vi "R5_Control.vi"() -> ()   [LabVIEW 2016]
uses:
  LabviewBioreactor/Reactor Control/R3R4/R2 example/R2 DO Manual Control.ctl
  LabviewBioreactor/Reactor Control/R3R4/R2 example/R2 Pump Manual Control.ctl
  LabviewBioreactor/Reactor Control/R3R4/R2 example/R2 pH Manual Control.ctl
  LabviewBioreactor/Reactor Control/R3R4/R2 example/R2 Reactor Status v1.ctl
  LabviewBioreactor/Reactor Control/R3R4/R2 example/R2Variables.lvlib
  LabviewBioreactor/Reactor Control/R3R4/R2 example/R2 SBR Mode Control.ctl
  R2 example/R2 Cycle Status.ctl
panel:
  out "Elapsed Time":dbl
  in  "Aerobic DO Control":T1={"DO set point (mg/L)"=2.0, "N2 Gain"=35.0, "Air Gain"=15.0, "DO Tolerance (mg/L)"=0.1, "Air Short Reaction Time (s)"=60.0, "Long Reaction Time (s)"=90.0, "N2 Short Reaction Time (s) 2"=15.0}
  out "pH and DO":cluster{"pH":dbl, "DO (mg/L)":dbl}(graph)
  out "DO Intercept":dbl
  out "DO Slope":dbl
  out "pH Intercept":dbl
  out "pH Slope":dbl
  in  "DO Control":T2
  in  "Reactor 2 Pumps Manual Control":T3
  in  "pH Control":T4
  in  "pH Control":T5={" pH Set Point"=7.5, " pH Tolerance"=0.1, "Reaction Time (s)"=15.0, "Pump On Time (s)"=3.0}
  out "Cycle Phase":T6 max=5.0 scale=0.0..160.0
  in  "SBR Timing":T7={"Anaerobic Time (min)"=60.0, "Aerobic (min)"=240.0, "Settle 1"=3.0, "Decant 1 (min)"=5.0, "Mix 2"=0.0, "Idle Time (min)"=5.0, "Aerobic no DO control (min)"=2.0, "Settle 2 (min)"=0.0, "Decant 2 (min)"=0.0, "Mix 3"=0.0, "Settle 3"=0.0, "Decant 3"=0.0}
  out "N2 and Air Flow":cluster{"N2 Flow":dbl, "Air Flow":dbl}(graph)
  out "Reactor 2 Status":T8 {"Compressed Air" format="%#.0g"; "Release Flow" format="%#.0g"; "DO Amp (A)" format="%#.4g"; "pH Amp (A)" format="%#.4g"; "DO (mg/L)" format="%#.2g"; "pH" format="%#.2g"}
  in  "Pumps Manual Control":bool
  in  "DO Manual Control":bool
  in  "pH Manual Control":bool=TRUE
  in  "DO Calibrate":bool
  in  "pH Calibrate":bool
  # "On: Manual Mode\nOff: SBR Mode"
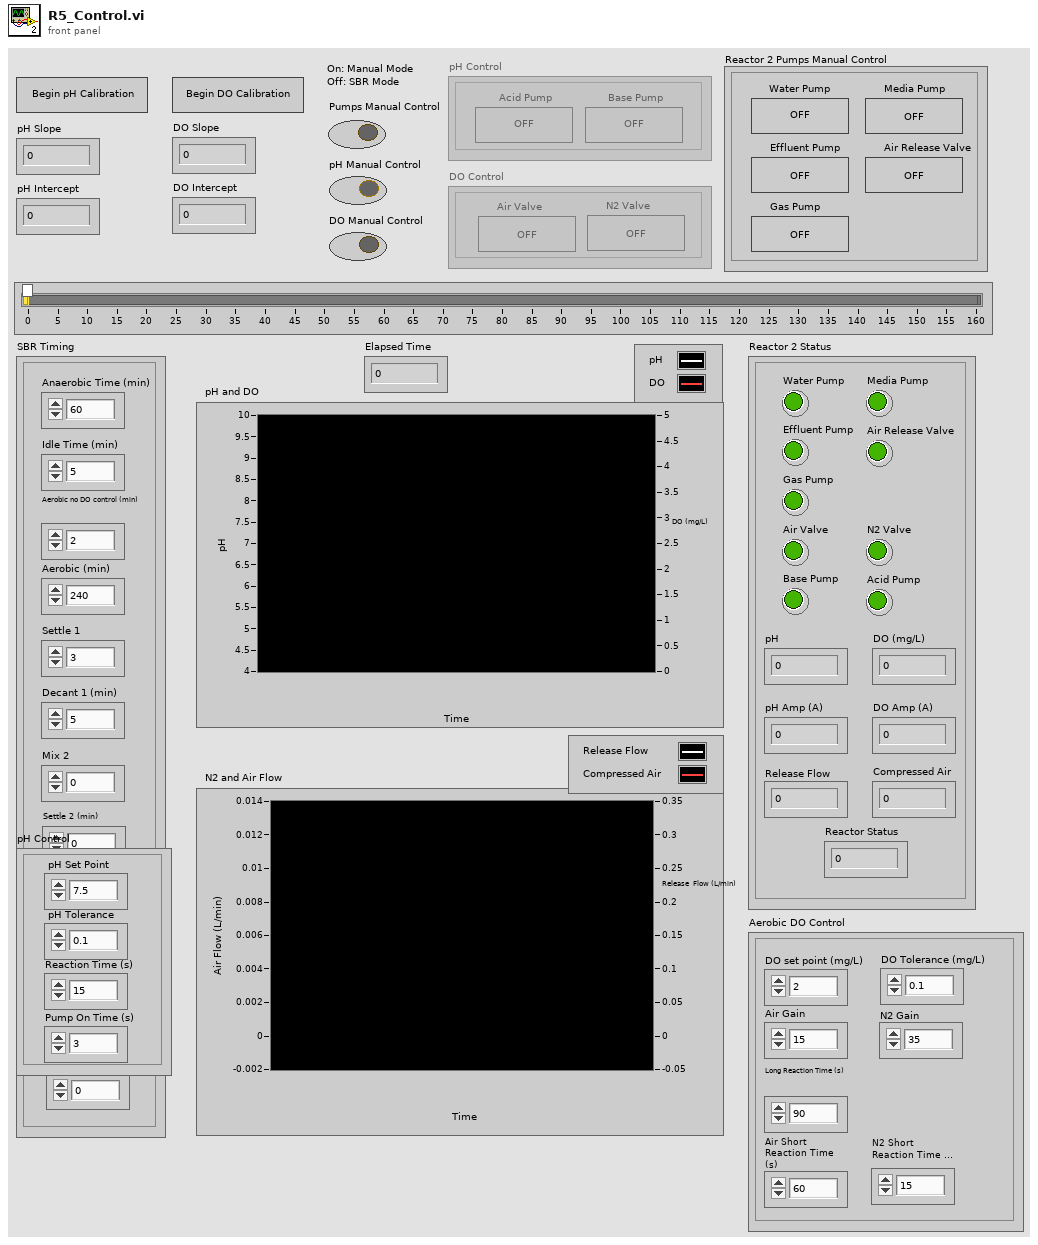
[diagram p1: front panel]
types:
  T1 = cluster{"DO set point (mg/L)":dbl, "N2 Gain":dbl, "Air Gain":dbl, "DO Tolerance (mg/L)":dbl, "Air Short Reaction Time (s)":dbl, "Long Reaction Time (s)":dbl, "N2 Short Reaction Time (s) 2":dbl}
  T2 = typedef "R2 DO Manual Control.ctl" = cluster{"Air Valve":bool, "N2 Valve":bool}
  T3 = typedef "R2Variables.lvlib/R2 Pump Manual Control.ctl" = cluster{"Water Pump":bool, "Effluent Pump":bool, "Media Pump":bool, "Gas Pump":bool, "Air Release Valve":bool}
  T4 = typedef "R2Variables.lvlib/R2 pH Manual Control.ctl" = cluster{"Acid Pump":bool, "Base Pump":bool}
  T5 = cluster{" pH Set Point":dbl, " pH Tolerance":dbl, "Reaction Time (s)":dbl, "Pump On Time (s)":dbl}
  T6 = typedef "R2Variables.lvlib/R2 Cycle Status.ctl" = dbl
  T7 = typedef "R2Variables.lvlib/R2 SBR Mode Control.ctl" = cluster{"Anaerobic Time (min)":dbl, "Aerobic (min)":dbl, "Settle 1":dbl, "Decant 1 (min)":dbl, "Mix 2":dbl, "Idle Time (min)":dbl, "Aerobic no DO control (min)":dbl, "Settle 2 (min)":dbl, "Decant 2 (min)":dbl, "Mix 3":dbl, "Settle 3":dbl, "Decant 3":dbl}
  T8 = typedef "R2Variables.lvlib/R2 Reactor Status v1.ctl" = cluster{"Water Pump":bool, "Media Pump":bool, "Effluent Pump":bool, "Base Pump":bool, "Gas Pump":bool, "Acid Pump":bool, "Air Release Valve":bool, "N2 Valve":bool, "pH":dbl, "DO (mg/L)":dbl, "pH Amp (A)":dbl, "DO Amp (A)":dbl, "Release Flow":dbl, "Compressed Air":dbl, "Reactor Status":sgl, "Air Valve":bool}
  T9 = enum8{"Enabled", "Disabled", "Disabled and Grayed Out"}
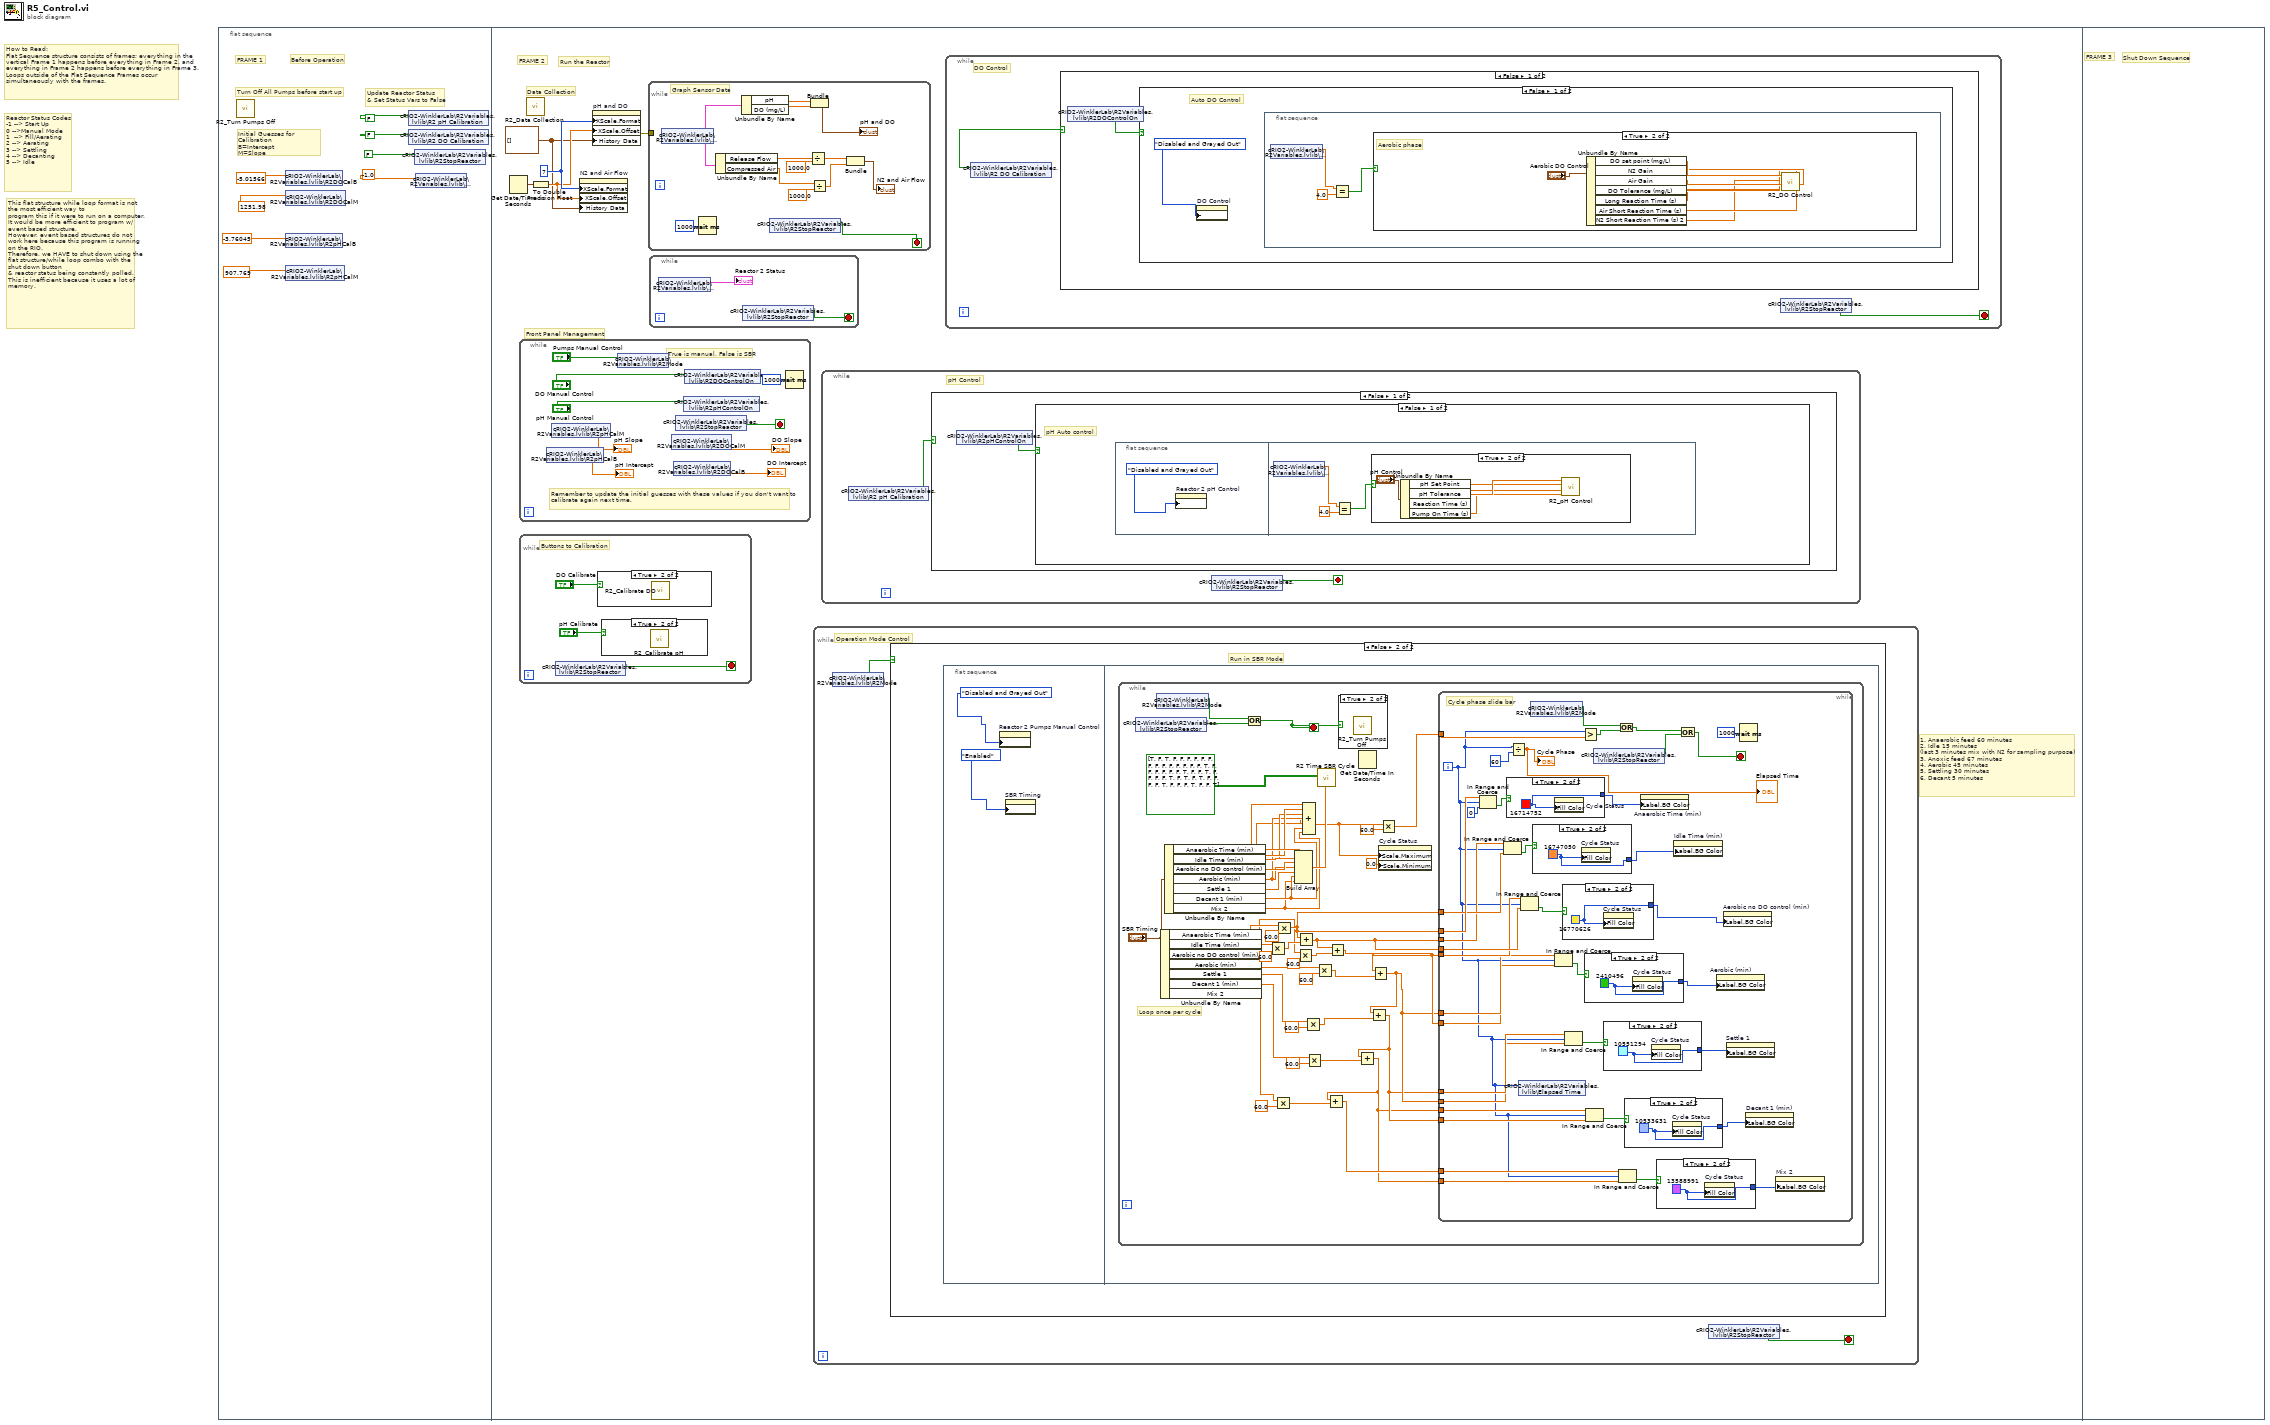
[diagram p0: block diagram]
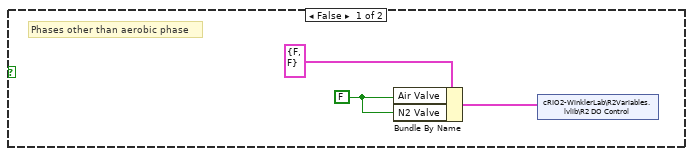
[diagram p2: hidden frame]
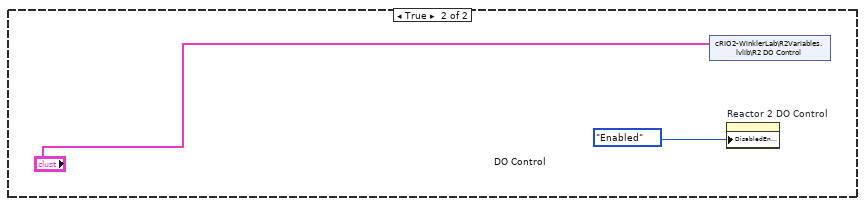
[diagram p3: hidden frame]
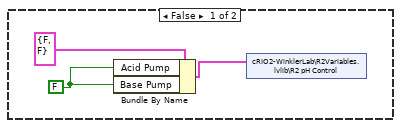
[diagram p7: hidden frame]
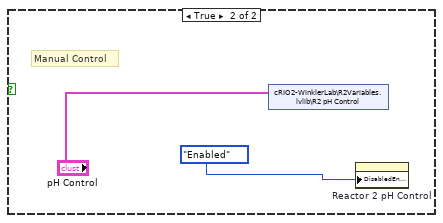
[diagram p8: hidden frame]
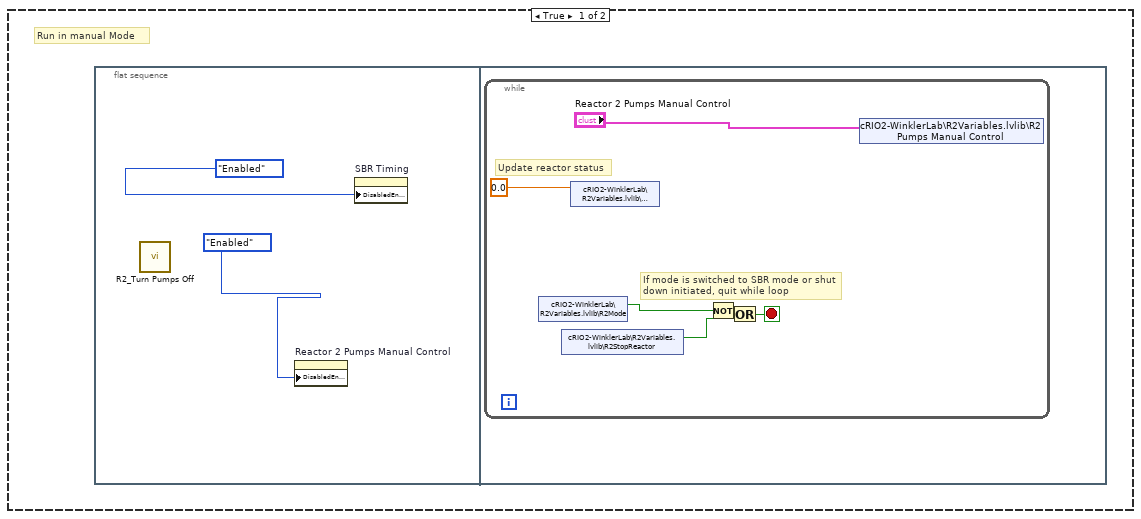
[diagram p10: hidden frame]
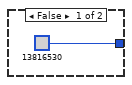
[diagram p11: hidden frame]
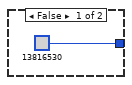
[diagram p12: hidden frame]
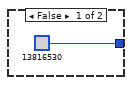
[diagram p13: hidden frame]
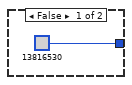
[diagram p14: hidden frame]
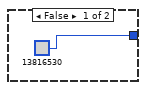
[diagram p15: hidden frame]
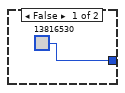
[diagram p16: hidden frame]
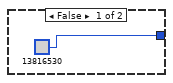
[diagram p17: hidden frame]
diagram:
  # "Reactor Status Codes\n-1 --> Start Up\n0 -->Manual Mode\n1  --> Fill/Aerating\n2 --> Aerating\n3 --> Settling\n4 --> Decanting\n5 --> Idle"
  # "How to Read:\nFlat Sequence structure consists of frames; everything in the vertical Frame 1 happens before everything in Frame 2, and everything in Frame 2 happens before everything in Frame 3.\nLoops outside of the Flat Sequence Frames occur simultaneously with the frames."
  # "This flat structure while loop format is not the most efficient way to \nprogram this if it were to run on a computer.\nIt would be more efficient to program w/ event based structure.\nHowever, event based structures do not work here because this program is running on the RIO.\nTherefore, we HAVE to shut down using the flat structure/while loop combo with the shut down button \n& reactor status being constantly polled.\nThis is inefficient because it uses a lot of memory."
  n1 = flat-sequence {
    frame #0 {
      # "Initial Guesses for Calibration\nB=Intercept\nM=Slope"
      # "Update Reactor Status \n& Set Status Vars to False"
      # "Turn Off All Pumps before start up"
      # "FRAME 1"
      # "Before Operation"
      n2 = call "R2_Turn Pumps Off.vi"() -> ()  [unwired: 12 in]
      n3 = shared-variable "cRIO2-WinklerLab\\R2Variables.lvlib\\R2DOCalB"(-5.01566 ("R1DOxCalB")) -> ()  [unwired: 1 in, 1 out]
      n4 = shared-variable "cRIO2-WinklerLab\\R2Variables.lvlib\\R2DOCalM"(1251.98 ("R1DOxCalM")) -> ()  [unwired: 1 in, 1 out]
      n5 = shared-variable "cRIO2-WinklerLab\\R2Variables.lvlib\\R2pHCalB"(-3.76045 ("R1pHCalB")) -> ()  [unwired: 1 in, 1 out]
      n6 = shared-variable "cRIO2-WinklerLab\\R2Variables.lvlib\\R2pHCalM"(907.769 ("R1pHCalM")) -> ()  [unwired: 1 in, 1 out]
      n7 = shared-variable "cRIO2-WinklerLab\\R2Variables.lvlib\\R2 pH Calibration"(FALSE ("pH Calibration")) -> ()  [unwired: 1 in, 1 out]
      n8 = shared-variable "cRIO2-WinklerLab\\R2Variables.lvlib\\R2 DO Calibration"(FALSE ("DO Calibration")) -> ()  [unwired: 1 in, 1 out]
      n9 = shared-variable "cRIO2-WinklerLab\\R2Variables.lvlib\\R2StopReactor"(FALSE ("R1Stop Reactor")) -> ()  [unwired: 1 in, 1 out]
      n10 = shared-variable "cRIO2-WinklerLab\\R2Variables.lvlib\\R2Phase"(-1.0) -> ()  [unwired: 1 in, 1 out]
    }
    frame #1 {
      w9 = cluster{"pH":dbl, "DO (mg/L)":dbl}[] [] ("History Data")
      w11 = u8 7 ("X Scale.Display Format:Format")
      # "1. Anaerobic feed 60 minutes\n2. Idle 15 minutes \n(last 3 minutes mix with N2 for sampling purpose)\n3. Anoxic feed 67 minutes\n4. Aerobic 45 minutes\n5. Settling 30 minutes\n6. Decant 5 minutes"
      # "Front Panel Management"
      # "Data Collection"
      # "FRAME 2"
      # "Run the Reactor"
      n11 = Get Date/Time In Seconds() -> (seconds since 1Jan1904=w13:timestamp)
      n12 = while {
        stop <- w73 stop-if-true
        # "Remember to update the initial guesses with these values if you don't want to calibrate again next time."
        # "True is manual, False is SBR"
        n13 = shared-variable "cRIO2-WinklerLab\\R2Variables.lvlib\\R2pHCalB"() -> (→"pH Intercept":dbl)  [unwired: 1 in, 1 out]
        n14 = shared-variable "cRIO2-WinklerLab\\R2Variables.lvlib\\R2pHCalM"() -> (→"pH Slope":dbl)  [unwired: 1 in, 1 out]
        n15 = shared-variable "cRIO2-WinklerLab\\R2Variables.lvlib\\R2Mode"("Pumps Manual Control") -> ()  [unwired: 1 in, 1 out]
        n16 = shared-variable "cRIO2-WinklerLab\\R2Variables.lvlib\\R2DOCalM"() -> (→"DO Slope":dbl)  [unwired: 1 in, 1 out]
        n17 = shared-variable "cRIO2-WinklerLab\\R2Variables.lvlib\\R2DOCalB"() -> (→"DO Intercept":dbl)  [unwired: 1 in, 1 out]
        n18 = shared-variable "cRIO2-WinklerLab\\R2Variables.lvlib\\R2StopReactor"() -> (w73:bool)  [unwired: 1 in, 1 out]
        n19 = shared-variable "cRIO2-WinklerLab\\R2Variables.lvlib\\R2pHControlOn"("pH Manual Control") -> ()  [unwired: 1 in, 1 out]
        n20 = shared-variable "cRIO2-WinklerLab\\R2Variables.lvlib\\R2DOControlOn"("DO Manual Control") -> ()  [unwired: 1 in, 1 out]
        n21 = Wait (ms)(milliseconds to wait=u32 1000) -> ()  [unwired: 1 out]
      }
      n22 = while {
        stop <- w49 stop-if-true
        # "Buttons to Calibration"
        n23 = shared-variable "cRIO2-WinklerLab\\R2Variables.lvlib\\R2StopReactor"() -> (w49:bool)  [unwired: 1 in, 1 out]
        n24 = case shown="True" "DO Calibrate" {
          frame False {
          }
          frame True {
            n25 = call "R2_Calibrate DO.vi"() -> ()  [unwired: 12 in]
          }
        }
        n26 = case shown="True" "pH Calibrate" {
          frame False {
          }
          frame True {
            n27 = call "R2_Calibrate pH.vi"() -> ()  [unwired: 12 in]
          }
        }
      }
      n28 = call "R2_Data Collection.vi"() -> ()  [unwired: 12 in]
      n29 = To Double Precision Float(number=w13) -> (double precision float=w10:dbl)
      n30 = property on="N2 and Air Flow" class="WFChart (strict)"("XScale.Format"=w11, "XScale.Offset"=w10, "History Data"=w9) -> ()  [unwired: 2 in, 2 out]
      n31 = property on="pH and DO" class="WFChart (strict)"("XScale.Format"=w11, "XScale.Offset"=w10, "History Data"=w9) -> (error out=w12:errorcluster)  [unwired: 2 in, 1 out]
      n32 = while {
        tunnel: w12 -> [_]
        stop <- w24 stop-if-true
        # "Graph Sensor Data"
        n33 = shared-variable "cRIO2-WinklerLab\\R2Variables.lvlib\\R2Status"() -> (w25:T8)  [unwired: 1 in, 1 out]
        n34 = Wait (ms)(milliseconds to wait=u32 1000) -> ()  [unwired: 1 out]
        n35 = Unbundle By Name(w25) -> ("Release Flow"=w21:dbl, "Compressed Air"=w18:dbl)
        n36 = Unbundle By Name(w25) -> ("pH"=w26:dbl, "DO (mg/L)"=w27:dbl)
        n37 = shared-variable "cRIO2-WinklerLab\\R2Variables.lvlib\\R2StopReactor"() -> (w24:bool)  [unwired: 1 in, 1 out]
        n38 = Divide(x=w21, y=1000.0) -> (x/y=w17:dbl)
        n39 = Bundle("pH"=w26, "DO (mg/L)"=w27) -> (→"pH and DO":cluster{"pH":dbl, "DO (mg/L)":dbl})  [unwired: 1 in]
        n40 = Divide(x=w18, y=1000.0) -> (x/y=w16:dbl)
        n41 = Bundle(w17, w16) -> (→"N2 and Air Flow":cluster{dbl, dbl})  [unwired: 1 in]
      }
      n42 = while {
        stop <- w14 stop-if-true
        n43 = shared-variable "cRIO2-WinklerLab\\R2Variables.lvlib\\R2Status"() -> (→"Reactor 2 Status":T8)  [unwired: 1 in, 1 out]
        n44 = shared-variable "cRIO2-WinklerLab\\R2Variables.lvlib\\R2StopReactor"() -> (w14:bool)  [unwired: 1 in, 1 out]
      }
      n45 = while {
        stop <- w79 stop-if-true
        # "Operation Mode Control"
        n46 = shared-variable "cRIO2-WinklerLab\\R2Variables.lvlib\\R2Mode"() -> (w78:bool)  [unwired: 1 in, 1 out]
        n47 = case shown="False" w78 {
          frame True {
            # "Run in manual Mode"
            n48 = flat-sequence {
              frame #0 {
                n49 = call "R2_Turn Pumps Off.vi"() -> ()  [unwired: 12 in]
                n50 = property on="Reactor 2 Pumps Manual Control" class="Clust (strict)"("DisabledEnum"=T9."Enabled" ("Disabled")) -> ()  [unwired: 2 in, 2 out]
                n51 = property on="SBR Timing" class="Clust (strict)"("DisabledEnum"=T9."Enabled" ("Disabled")) -> ()  [unwired: 2 in, 2 out]
              }
              frame #1 {
                n52 = while {
                  stop <- w86 stop-if-true
                  # "If mode is switched to SBR mode or shut \ndown initiated, quit while loop"
                  # "Update reactor status"
                  n53 = shared-variable "cRIO2-WinklerLab\\R2Variables.lvlib\\R2Mode"() -> (w84:bool)  [unwired: 1 in, 1 out]
                  n54 = shared-variable "cRIO2-WinklerLab\\R2Variables.lvlib\\R2StopReactor"() -> (w83:bool)  [unwired: 1 in, 1 out]
                  n55 = shared-variable "cRIO2-WinklerLab\\R2Variables.lvlib\\R2Phase"(0.0 ("Reactor Status")) -> ()  [unwired: 1 in, 1 out]
                  n56 = Not(x=w84) -> (.not. x?=w87:bool)
                  n57 = Or(x=w87, y=w83) -> (x .or. y?=w86:bool)
                  n58 = shared-variable "cRIO2-WinklerLab\\R2Variables.lvlib\\R2 Pumps Manual Control"("Reactor 2 Pumps Manual Control") -> ()  [unwired: 1 in, 1 out]
                }
              }
            }
          }
          frame False {
            # "Run in SBR Mode"
            n59 = flat-sequence {
              frame #0 {
                n60 = property on="Reactor 2 Pumps Manual Control" class="Clust (strict)"("DisabledEnum"=T9."Disabled and Grayed Out" ("Disabled")) -> ()  [unwired: 2 in, 2 out]
                n61 = property on="SBR Timing" class="Clust (strict)"("DisabledEnum"=T9."Enabled" ("Disabled")) -> ()  [unwired: 2 in, 2 out]
              }
              frame #1 {
                n62 = while {
                  stop <- w133 stop-if-true
                  # "Loop once per cycle"
                  n63 = shared-variable "cRIO2-WinklerLab\\R2Variables.lvlib\\R2StopReactor"() -> (w131:bool)  [unwired: 1 in, 1 out]
                  n64 = shared-variable "cRIO2-WinklerLab\\R2Variables.lvlib\\R2Mode"() -> (w132:bool)  [unwired: 1 in, 1 out]
                  n65 = Unbundle By Name("SBR Timing") -> ("Anaerobic Time (min)"=w118:dbl, "Idle Time (min)"=w113:dbl, "Aerobic no DO control (min)"=w111:dbl, "Aerobic (min)"=w109:dbl, "Settle 1"=w105:dbl, "Decant 1 (min)"=w98:dbl, "Mix 2"=w93:dbl)
                  n66 = Unbundle By Name("SBR Timing") -> ("Anaerobic Time (min)"=w129:dbl, "Idle Time (min)"=w128:dbl, "Aerobic no DO control (min)"=w127:dbl, "Aerobic (min)"=w126:dbl, "Settle 1"=w125:dbl, "Decant 1 (min)"=w100:dbl, "Mix 2"=w90:dbl)
                  n67 = Or(x=w132, y=w131) -> (x .or. y?=w133:bool)
                  n68 = Multiply(x=w113, y=60.0) -> (x*y=w112:dbl)
                  n69 = Multiply(x=w93, y=60.0) -> (x*y=w94:dbl)
                  n70 = Multiply(x=w118, y=60.0) -> (x*y=w117:dbl)
                  n71 = Build Array(w129, w128, w127, w126, w125, w100, w90) -> (w124:dbl[])
                  n72 = Multiply(x=w111, y=60.0) -> (x*y=w110:dbl)
                  n73 = Add(x=w117, y=w112) -> (x+y=w119:dbl)
                  n74 = Compound Arithmetic op=ADD(w129, w128, w127, w126, w125, w100, w90) -> (w120:dbl)
                  n75 = Multiply(x=w105, y=60.0) -> (x*y=w104:dbl)
                  n76 = Multiply(x=w98, y=60.0) -> (x*y=w97:dbl)
                  n77 = Multiply(x=w109, y=60.0) -> (x*y=w103:dbl)
                  n78 = call "R2 Time SBR Cycle.vi"("Pump Status Array"=bool[][] [[TRUE, FALSE, TRUE, FALSE, FALSE, FALSE, FALSE], [FALSE, FALSE, FALSE, FALSE, FALSE, FALSE, FALSE], [FALSE, FALSE, FALSE, TRUE, FALSE, FALSE, FALSE], [FALSE, FALSE, FALSE, TRUE, FALSE, FALSE, TRUE], [FALSE, FALSE, FALSE, FALSE, TRUE, FALSE, TRUE], [FALSE, TRUE, FALSE, FALSE, FALSE, FALSE, TRUE], [FALSE, FALSE, FALSE, TRUE, FALSE, FALSE, TRUE]], "Timing Array"=w124) -> ()  [unwired: 10 in]
                  n79 = Add(x=w119, y=w110) -> (x+y=w102:dbl)
                  n80 = case shown="True" w133 {
                    frame False {
                    }
                    frame True {
                      n81 = call "R2_Turn Pumps Off.vi"() -> ()  [unwired: 12 in]
                    }
                  }
                  n82 = Get Date/Time In Seconds() -> ()  [unwired: 1 out]
                  n83 = Add(x=w102, y=w103) -> (x+y=w101:dbl)
                  n84 = Add(x=w101, y=w104) -> (x+y=w96:dbl)
                  n85 = Add(x=w96, y=w97) -> (x+y=w91:dbl)
                  n86 = Add(x=w91, y=w94) -> (x+y=w92:dbl)
                  n87 = property on="Cycle Status" class="Slide (strict)"("Scale.Maximum"=w120, "Scale.Minimum"=0.0 ("Scale.Range:Minimum")) -> ()  [unwired: 2 in, 2 out]
                  n88 = Multiply(x=w120, y=60.0) -> (x*y=w121:dbl)
                  n89 = while {
                    tunnel: w121 -> [w170]
                    tunnel: w117 -> [w165]
                    tunnel: w117 -> [w162]
                    tunnel: w119 -> [w161]
                    tunnel: w119 -> [w160]
                    tunnel: w102 -> [w159]
                    tunnel: w101 -> [w158]
                    tunnel: w96 -> [w151]
                    tunnel: w101 -> [w150]
                    tunnel: w102 -> [w148]
                    tunnel: w91 -> [w146]
                    tunnel: w96 -> [w145]
                    tunnel: w92 -> [w143]
                    tunnel: w91 -> [w142]
                    i -> [w141]
                    stop <- w152 stop-if-true
                    # "Cycle phase slide bar"
                    n90 = In Range and Coerce(upper limit=w165, x=w141, lower limit=0) -> (In Range?=w168:bool)  [unwired: 1 out]
                    n91 = In Range and Coerce(upper limit=w161, x=w141, lower limit=w162) -> (In Range?=w166:bool)  [unwired: 1 out]
                    n92 = case shown="True" w168 {
                      tunnel: [u32 13816530 w185] -> w157
                      frame False {
                      }
                      frame True {
                        w185 = u32 16714752
                        n93 = property on="Cycle Status" class="Slide (strict)"("Fill Color"=w185) -> ()  [unwired: 2 in, 2 out]
                      }
                    }
                    n94 = Divide(x=w141, y=60) -> (x/y=→"Cycle Phase" →"Elapsed Time":dbl)
                    n95 = shared-variable "cRIO2-WinklerLab\\R2Variables.lvlib\\Elapsed Time"(w141) -> ()  [unwired: 1 in, 1 out]
                    n96 = In Range and Coerce(upper limit=w159, x=w141, lower limit=w160) -> (In Range?=w164:bool)  [unwired: 1 out]
                    n97 = shared-variable "cRIO2-WinklerLab\\R2Variables.lvlib\\R2Mode"() -> (w155:bool)  [unwired: 1 in, 1 out]
                    n98 = case shown="True" w166 {
                      tunnel: [u32 13816530 w183] -> w140
                      frame False {
                      }
                      frame True {
                        w183 = u32 16747050
                        n99 = property on="Cycle Status" class="Slide (strict)"("Fill Color"=w183) -> ()  [unwired: 2 in, 2 out]
                      }
                    }
                    n100 = In Range and Coerce(upper limit=w158, x=w141, lower limit=w148) -> (In Range?=w163:bool)  [unwired: 1 out]
                    n101 = case shown="True" w164 {
                      tunnel: [u32 13816530 w181] -> w135
                      frame False {
                      }
                      frame True {
                        w181 = u32 16770626
                        n102 = property on="Cycle Status" class="Slide (strict)"("Fill Color"=w181) -> ()  [unwired: 2 in, 2 out]
                      }
                    }
                    n103 = In Range and Coerce(upper limit=w151, x=w141, lower limit=w150) -> (In Range?=w149:bool)  [unwired: 1 out]
                    n104 = Greater?(x=w141, y=w170) -> (0:w156:bool)
                    n105 = case shown="True" w163 {
                      tunnel: [u32 13816530 w179] -> w139
                      frame False {
                      }
                      frame True {
                        w179 = u32 2410496
                        n106 = property on="Cycle Status" class="Slide (strict)"("Fill Color"=w179) -> ()  [unwired: 2 in, 2 out]
                      }
                    }
                    n107 = In Range and Coerce(upper limit=w146, x=w141, lower limit=w145) -> (In Range?=w147:bool)  [unwired: 1 out]
                    n108 = shared-variable "cRIO2-WinklerLab\\R2Variables.lvlib\\R2StopReactor"() -> (w153:bool)  [unwired: 1 in, 1 out]
                    n109 = case shown="True" w149 {
                      tunnel: [u32 13816530 w177] -> w138
                      frame False {
                      }
                      frame True {
                        w177 = u32 10551294
                        n110 = property on="Cycle Status" class="Slide (strict)"("Fill Color"=w177) -> ()  [unwired: 2 in, 2 out]
                      }
                    }
                    n111 = Or(x=w155, y=w156) -> (x .or. y?=w154:bool)
                    n112 = In Range and Coerce(upper limit=w143, x=w141, lower limit=w142) -> (In Range?=w144:bool)  [unwired: 1 out]
                    n113 = case shown="True" w147 {
                      tunnel: [u32 13816530 w175] -> w137
                      frame False {
                      }
                      frame True {
                        w175 = u32 10533631
                        n114 = property on="Cycle Status" class="Slide (strict)"("Fill Color"=w175) -> ()  [unwired: 2 in, 2 out]
                      }
                    }
                    n115 = property on="Anaerobic Time (min)" class="DigNum (strict)"("Label.BG Color"=w157) -> ()  [unwired: 2 in, 2 out]
                    n116 = case shown="True" w144 {
                      tunnel: [u32 13816530 w173] -> w136
                      frame False {
                      }
                      frame True {
                        w173 = u32 13588991
                        n117 = property on="Cycle Status" class="Slide (strict)"("Fill Color"=w173) -> ()  [unwired: 2 in, 2 out]
                      }
                    }
                    n118 = property on="Idle Time (min)" class="DigNum (strict)"("Label.BG Color"=w140) -> ()  [unwired: 2 in, 2 out]
                    n119 = Or(x=w154, y=w153) -> (x .or. y?=w152:bool)
                    n120 = property on="Aerobic (min)" class="DigNum (strict)"("Label.BG Color"=w139) -> ()  [unwired: 2 in, 2 out]
                    n121 = property on="Aerobic no DO control (min)" class="DigNum (strict)"("Label.BG Color"=w135) -> ()  [unwired: 2 in, 2 out]
                    n122 = property on="Settle 1" class="DigNum (strict)"("Label.BG Color"=w138) -> ()  [unwired: 2 in, 2 out]
                    n123 = Wait (ms)(milliseconds to wait=u32 1000) -> ()  [unwired: 1 out]
                    n124 = property on="Decant 1 (min)" class="DigNum (strict)"("Label.BG Color"=w137) -> ()  [unwired: 2 in, 2 out]
                    n125 = property on="Mix 2" class="DigNum (strict)"("Label.BG Color"=w136) -> ()  [unwired: 2 in, 2 out]
                  }
                }
              }
            }
          }
        }
        n126 = shared-variable "cRIO2-WinklerLab\\R2Variables.lvlib\\R2StopReactor"() -> (w79:bool)  [unwired: 1 in, 1 out]
      }
      n127 = while {
        stop <- w53 stop-if-true
        # "pH Control"
        n128 = shared-variable "cRIO2-WinklerLab\\R2Variables.lvlib\\R2 pH Calibration"() -> (w52:bool)  [unwired: 1 in, 1 out]
        n129 = case shown="False" w52 {
          frame False {
            n130 = shared-variable "cRIO2-WinklerLab\\R2Variables.lvlib\\R2pHControlOn"() -> (w54:bool)  [unwired: 1 in, 1 out]
            n131 = case shown="False" w54 {
              frame False {
                # "pH Auto control"
                n132 = flat-sequence {
                  frame #0 {
                    n133 = property on="Reactor 2 pH Control" class="Clust (strict)"("DisabledEnum"=T9."Disabled and Grayed Out" ("Disabled")) -> ()  [unwired: 2 in, 2 out]
                  }
                  frame #1 {
                    n134 = shared-variable "cRIO2-WinklerLab\\R2Variables.lvlib\\R2Phase"() -> (w58:dbl)  [unwired: 1 in, 1 out]
                    n135 = Equal?(x=w58, y=4.0) -> (x = y?=w56:bool)
                    n136 = case shown="True" w56 {
                      frame False {
                        w60 = FALSE
                        n137 = Bundle By Name(cluster=T4 {"Acid Pump"=FALSE, "Base Pump"=FALSE} ("Reactor 2 pH Control"), "Acid Pump"=w60, "Base Pump"=w60) -> (w59:T4)
                        n138 = shared-variable "cRIO2-WinklerLab\\R2Variables.lvlib\\R2 pH Control"(w59) -> ()  [unwired: 1 in, 1 out]
                      }
                      frame True {
                        n139 = Unbundle By Name("pH Control") -> ("pH Set Point"=w64:dbl, "pH Tolerance"=w65:dbl, "Reaction Time (s)"=w63:dbl, "Pump On Time (s)"=w62:dbl)
                        n140 = call "R2_pH Control.vi"("Pump On Time (s)"=w62, "Reaction Time (s)"=w63, "pH Set Point"=w64, "pH Tolerance"=w65) -> ()  [unwired: 8 in]
                      }
                    }
                  }
                }
              }
              frame True {
                # "Manual Control"
                n141 = shared-variable "cRIO2-WinklerLab\\R2Variables.lvlib\\R2 pH Control"("pH Control") -> ()  [unwired: 1 in, 1 out]
                n142 = property on="Reactor 2 pH Control" class="Clust (strict)"("DisabledEnum"=T9."Enabled" ("Disabled")) -> ()  [unwired: 2 in, 2 out]
              }
            }
          }
          frame True {
          }
        }
        n143 = shared-variable "cRIO2-WinklerLab\\R2Variables.lvlib\\R2StopReactor"() -> (w53:bool)  [unwired: 1 in, 1 out]
      }
      n144 = while {
        stop <- w30 stop-if-true
        # "DO Control"
        n145 = shared-variable "cRIO2-WinklerLab\\R2Variables.lvlib\\R2 DO Calibration"() -> (w29:bool)  [unwired: 1 in, 1 out]
        n146 = case shown="False" w29 {
          frame False {
            n147 = shared-variable "cRIO2-WinklerLab\\R2Variables.lvlib\\R2DOControlOn"() -> (w31:bool)  [unwired: 1 in, 1 out]
            n148 = case shown="False" w31 {
              frame False {
                # "Auto DO Control"
                n149 = property on="DO Control" class="Clust (strict)"("DisabledEnum"=T9."Disabled and Grayed Out" ("Disabled")) -> ()  [unwired: 2 in, 2 out]
                n150 = flat-sequence {
                  frame #0 {
                    n151 = shared-variable "cRIO2-WinklerLab\\R2Variables.lvlib\\R2Phase"() -> (w35:dbl)  [unwired: 1 in, 1 out]
                    n152 = Equal?(x=w35, y=4.0) -> (x = y?=w33:bool)
                    n153 = case shown="True" w33 {
                      frame False {
                        w37 = FALSE
                        # "Phases other than aerobic phase"
                        n154 = Bundle By Name(cluster=T2 {"Air Valve"=FALSE, "N2 Valve"=FALSE} ("Reactor 2 DO Control"), "Air Valve"=w37, "N2 Valve"=w37) -> (w38:T2)
                        n155 = shared-variable "cRIO2-WinklerLab\\R2Variables.lvlib\\R2 DO Control"(w38) -> ()  [unwired: 1 in, 1 out]
                      }
                      frame True {
                        # "Aerobic phase"
                        n156 = Unbundle By Name("Aerobic DO Control") -> ("DO set point (mg/L)"=w45:dbl, "N2 Gain"=w44:dbl, "Air Gain"=w43:dbl, "DO Tolerance (mg/L)"=w42:dbl, "Long Reaction Time (s)"=w41:dbl, "Air Short Reaction Time (s)"=w40:dbl, "N2 Short Reaction Time (s) 2"=w39:dbl)
                        n157 = call "R2_DO Control.vi"("Air Short Reaction Time (s)"=w40, "N2 Gain"=w44, "DO Tolerance (mg/L)"=w42, "Long Reaction Time (s)"=w41, "Air Gain"=w43, "N2 Short Reaction Time (s)"=w39, "DO Set Point (mg/L)"=w45) -> ()  [unwired: 1 in]
                      }
                    }
                  }
                }
              }
              frame True {
                n158 = shared-variable "cRIO2-WinklerLab\\R2Variables.lvlib\\R2 DO Control"("DO Control") -> ()  [unwired: 1 in, 1 out]
                n159 = property on="Reactor 2 DO Control" class="Clust (strict)"("DisabledEnum"=T9."Enabled" ("Disabled")) -> ()  [unwired: 2 in, 2 out]
              }
            }
          }
          frame True {
          }
        }
        n160 = shared-variable "cRIO2-WinklerLab\\R2Variables.lvlib\\R2StopReactor"() -> (w30:bool)  [unwired: 1 in, 1 out]
      }
    }
    frame #2 {
      # "FRAME 3"
      # "Shut Down Sequence"
    }
  }
